vi "Pick Device.vi"(1 "Max Devices":i32, 2 "Device Selected":bool[](array[boolean]), 3 "Available Devices:":string[][](array[string])) -> (0 "Return Address":string)   [LabVIEW 2011]
panel:
  in  "Cancel":bool
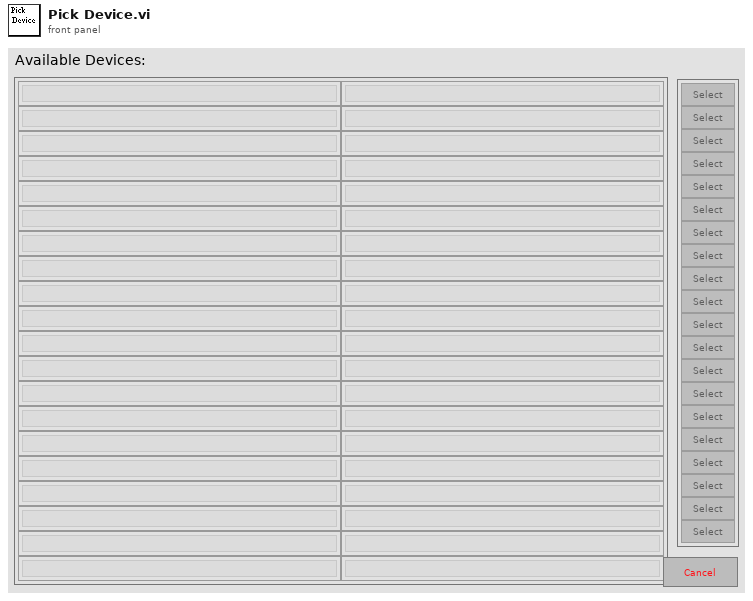
[diagram p1: front panel]
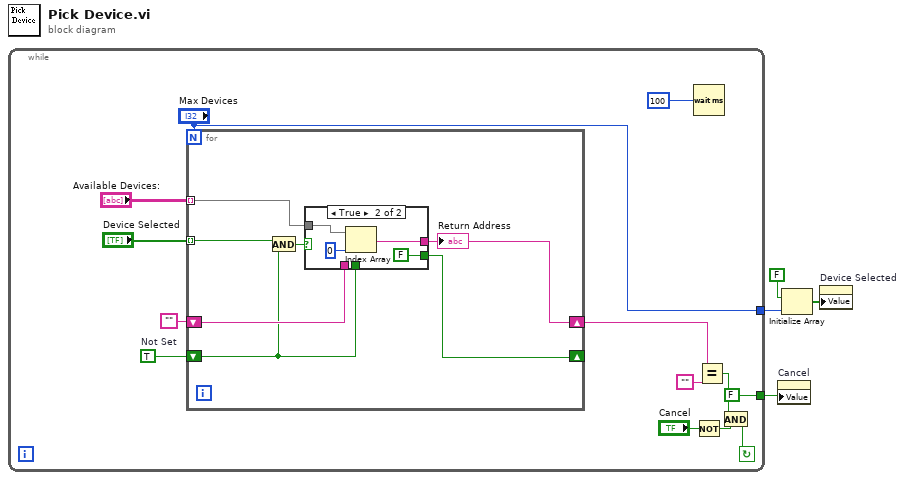
[diagram p0: block diagram]
diagram:
  n1 = while {
    tunnel: [FALSE] -> w1
    tunnel: ["Max Devices"] -> w3
    stop <- w9 continue-if-true
    w15 = TRUE  # Not Set
    n2 = for {
      N: "Max Devices" -> [_]
      tunnel: "Device Selected" -> [w22] mode=indexing
      tunnel: "Available Devices:" -> [w24] mode=indexing
      shift-right: [w21] -> _
      shift-left: w15 -> [w18]
      shift-right: [w19] -> w13
      shift-left: "" -> [w20]
      n3 = And(x=w22, y=w18) -> (x .and. y?=w23:bool)
      n4 = case shown="True" w23 {
        tunnel: [w26 w29] -> w19
        tunnel: w24 -> [_ w30]
        tunnel: [w25 FALSE] -> w21
        tunnel: w20 -> [w26 _]
        tunnel: w18 -> [w25 _]
        frame False {
        }
        frame True {
          n5 = Index Array(array=w30, index=0) -> (element=w29:string)
        }
      }
      "Return Address" <- w19
    }
    n6 = Wait (ms)(milliseconds to wait=100) -> ()  [unwired: 1 out]
    n7 = Not(x="Cancel") -> (.not. x?=w7:bool)
    n8 = Equal?(x=w13, y="") -> (x = y?=w10:bool)
    n9 = And(x=w10, y=w7) -> (x .and. y?=w9:bool)
  }
  n10 = property on="Cancel" class="Bool"("Value"=w1) -> ()  [unwired: 2 in, 2 out]
  n11 = Initialize Array(FALSE, w3) -> (w4:bool[])
  n12 = property on="Device Selected" class="Arr"("Value"=w4) -> ()  [unwired: 2 in, 2 out]
